vi "AI Test Temp serial v7.vi"(0 "Command String":string, 5 "Time Out (S)":dbl, 7 "CALIB":dbl) -> (4 "T1":dbl, 6 "T2":dbl, 8 "T3":dbl, 10 "T4":dbl, 13 "error":bool, 14 "output cluster":cluster{dbl, dbl, dbl, dbl, i32, "error #":dbl}, 15 "Unit ID":dbl)   [LabVIEW 2013]
panel:
  out "VISA Com out":refnum<visa-resource-name>
  out "Com Port Create loops":i32
  out "Com Port Create":bool
  in  "Select COM port":refnum<visa-resource-name>
  out "error out 1":errorcluster
  in  "Loop Time mS":u32
  in  "stop":bool
  out "error #":dbl
  out "End T":dbl
  out "Start T":dbl
  out "read time":dbl
  in  "Array - String":string[](array[string])
  out "end of data (#)":bool
  out "data bytes read":dbl
  out "data string":string
  out "read buffer":string
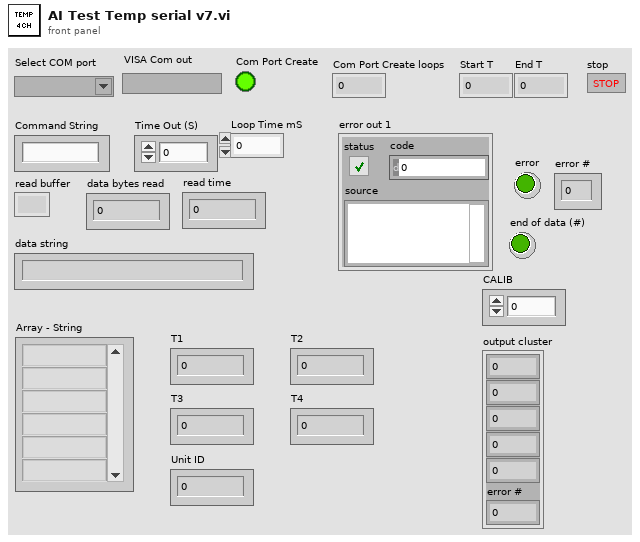
[diagram p1: front panel]
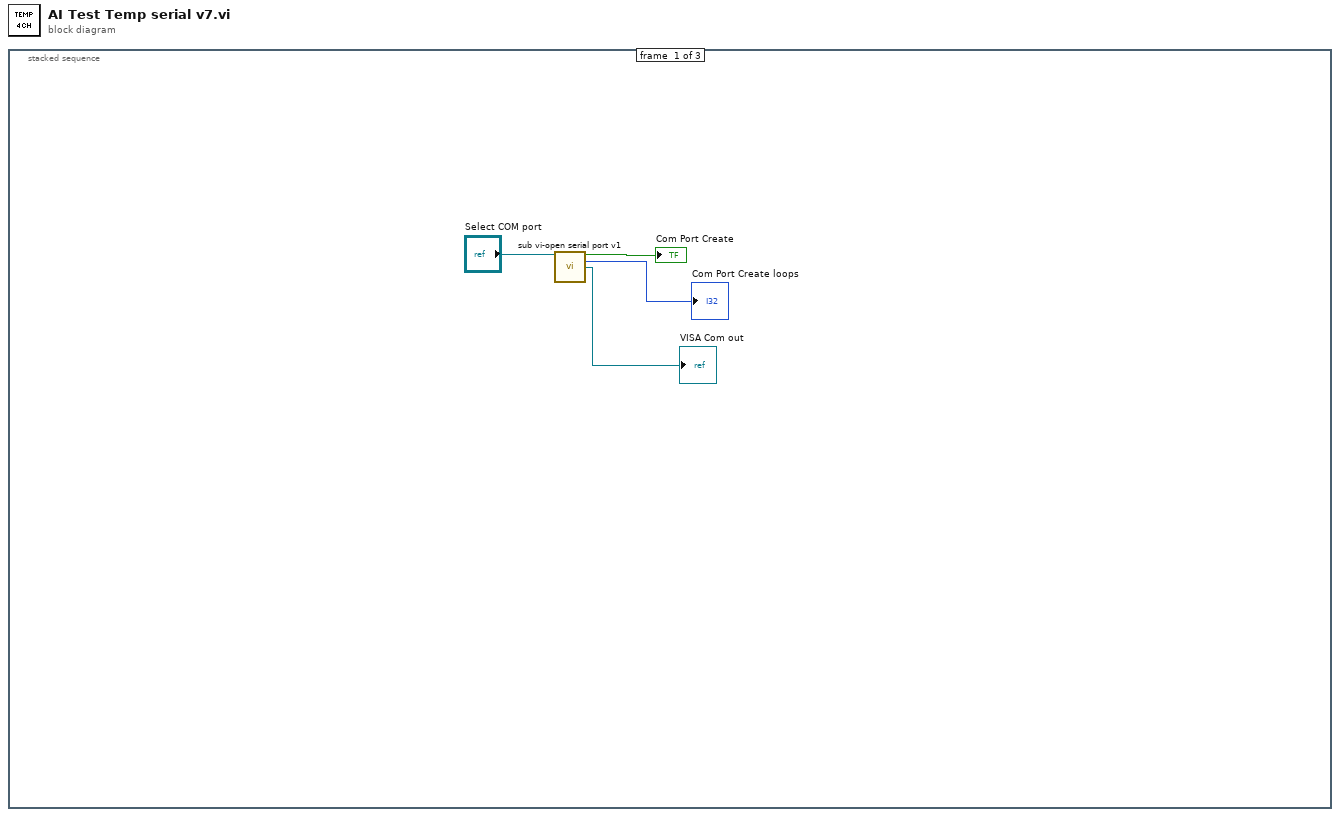
[diagram p0: block diagram]
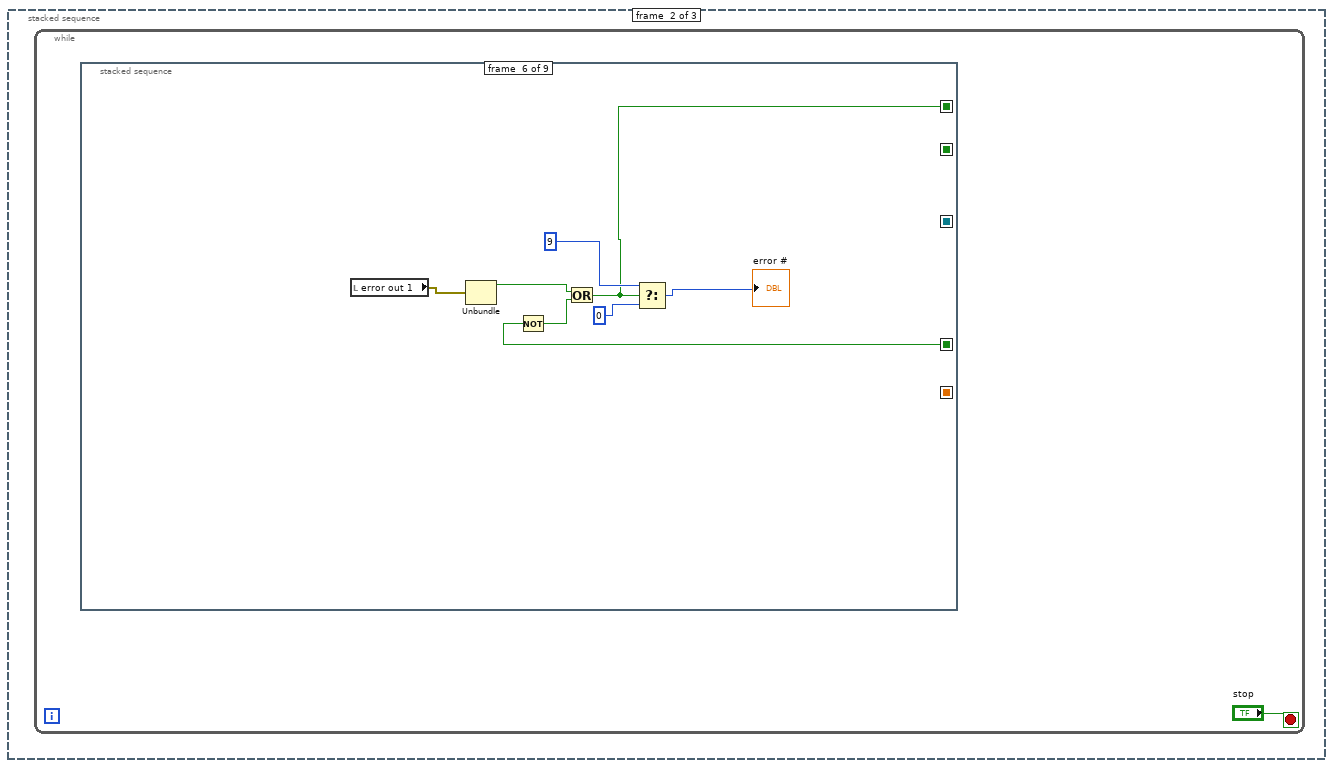
[diagram p2: hidden frame]
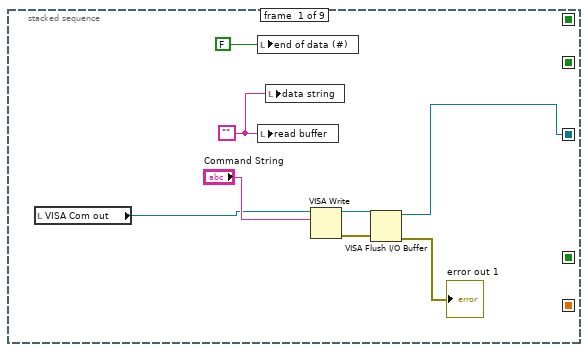
[diagram p3: hidden frame]
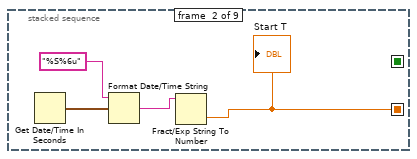
[diagram p4: hidden frame]
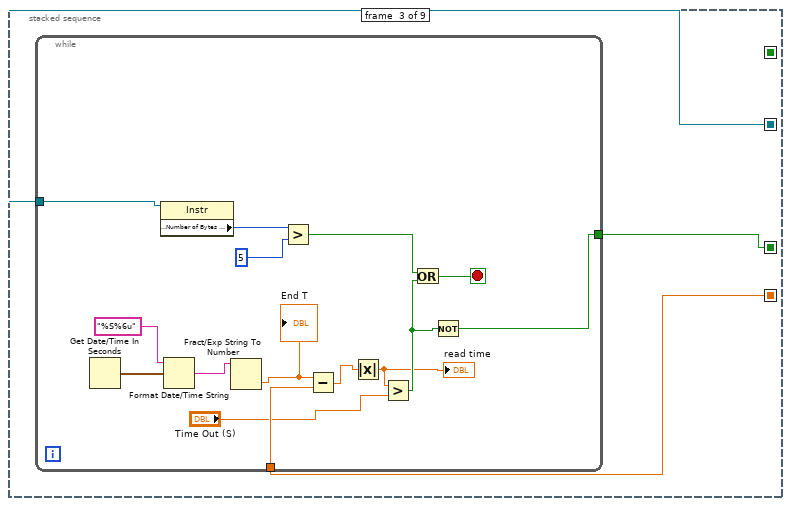
[diagram p5: hidden frame]
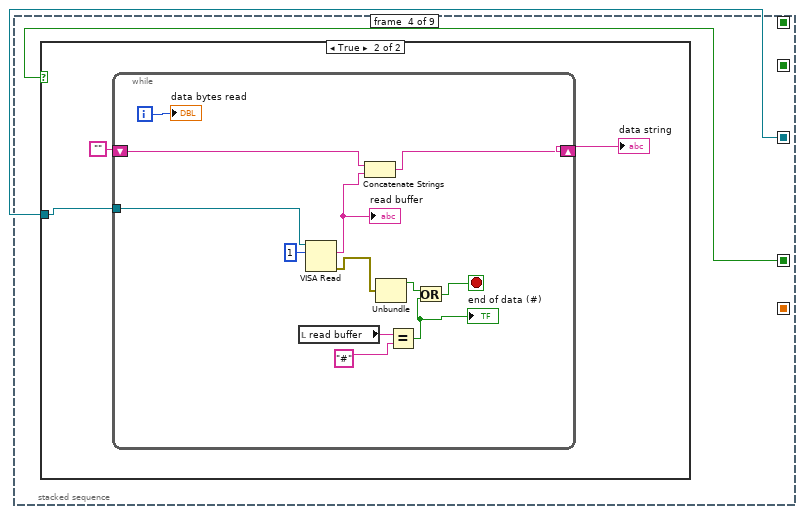
[diagram p6: hidden frame]
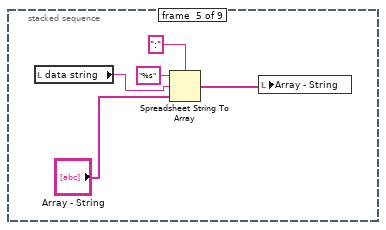
[diagram p8: hidden frame]
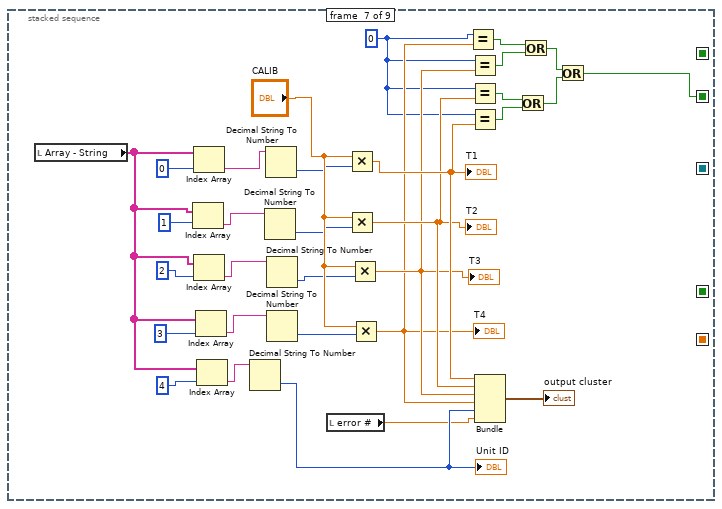
[diagram p9: hidden frame]
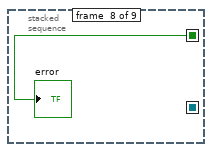
[diagram p10: hidden frame]
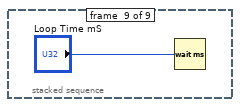
[diagram p11: hidden frame]
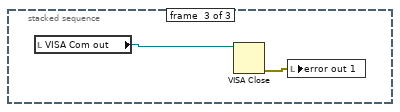
[diagram p12: hidden frame]
diagram:
  n1 = stacked-sequence {
    frame #0 {
      n2 = call "sub vi-open serial port v1.vi"("Select COM port"="Select COM port") -> ("status"=→"Com Port Create":bool, "LOOPS"=→"Com Port Create loops":i32, "VISA Com out"=→"VISA Com out":refnum<visa-resource-name>)  [unwired: 12 in]
    }
    frame #1 {
      n3 = while {
        stop <- "stop" stop-if-true
        n4 = stacked-sequence {
          seq-local: [_ _ w20 _ _ _ _ _ _] -> [_ _ _ w37 _ w65 _ _ _]
          seq-local: [_ w14 _ _ _ _ _ _ _] -> [_ _ w19 _ _ _ _ _ _]
          seq-local: [_ _ _ _ _ w60 _ _ _] -> [_ _ _ _ _ _ _ _ _]
          seq-local: [_ _ _ _ _ _ w66 _ _] -> [_ _ _ _ _ _ _ w97 _]
          seq-local: [w9 _ _ _ _ _ _ _ _] -> [_ _ w18 w36 _ _ _ _ _]
          frame #0 {
            w13 = ""
            n5 = local read "VISA Com out"() -> (w7:refnum<visa-resource-name>)
            n6 = local write "end of data (#)"(FALSE) -> ()
            n7 = local write "read buffer"(w13) -> ()
            n8 = local write "data string"(w13) -> ()
            n9 = VISA Write(VISA resource name=w7, write buffer="Command String") -> (VISA resource name out=w11:refnum<visa-resource-name>, error out=w6:errorcluster)  [unwired: 1 in, 1 out]
            n10 = VISA Flush I/O Buffer(VISA resource name=w11, error in (no error)=w6) -> (VISA resource name out=w9:refnum<visa-resource-name>, error out=→"error out 1":errorcluster)  [unwired: 1 in]
          }
          frame #1 {
            n11 = Get Date/Time In Seconds() -> (seconds since 1Jan1904=w17:timestamp)
            n12 = Format Date/Time String(time format string (%c)="%S%6u", seconds (now)=w17) -> (date/time string=w15:string)  [unwired: 1 in]
            n13 = Fract/Exp String To Number(string=w15) -> (number=w14:dbl)  [unwired: 3 in, 1 out]
            "Start T" <- w14
          }
          frame #2 {
            n14 = while {
              tunnel: w18 -> [w35]
              tunnel: [w24] -> w20
              tunnel: w19 -> [w28]
              stop <- w26 stop-if-true
              n15 = Get Date/Time In Seconds() -> (seconds since 1Jan1904=w32:timestamp)
              n16 = property class="Instr"(reference=w35) -> ("Serial Settings:Number of Bytes at Serial Port"=w34:u32)  [unwired: 1 in, 2 out]
              n17 = Format Date/Time String(time format string (%c)="%S%6u", seconds (now)=w32) -> (date/time string=w30:string)  [unwired: 1 in]
              n18 = Fract/Exp String To Number(string=w30) -> (number=w29:dbl)  [unwired: 3 in, 1 out]
              "End T" <- w29
              n19 = Greater?(x=w34, y=5) -> (0:w27:bool)
              n20 = Subtract(x=w29, y=w28) -> (x-y=w22:dbl)
              n21 = Absolute Value(x=w22) -> (abs(x)=w21:dbl)
              "read time" <- w21
              n22 = Greater?(x=w21, y="Time Out (S)") -> (0:w25:bool)
              n23 = Or(x=w27, y=w25) -> (x .or. y?=w26:bool)
              n24 = Not(x=w25) -> (.not. x?=w24:bool)
            }
          }
          frame #3 {
            n25 = case shown="True" w37 {
              tunnel: w36 -> [_ w40]
              frame False {
              }
              frame True {
                n26 = while {
                  tunnel: w40 -> [w47]
                  shift-right: [w46] -> w39
                  shift-left: "" -> [w45]
                  i -> [w48]
                  stop <- w41 stop-if-true
                  n27 = local read "read buffer"() -> (w51:string)
                  n28 = VISA Read(VISA resource name=w47, byte count=u32 1) -> (read buffer=w49:string, error out=w44:errorcluster)  [unwired: 1 in, 2 out]
                  "read buffer" <- w49
                  n29 = Concatenate Strings(w45, w49) -> (w46:string)
                  n30 = Unbundle(w44) -> ("status"=w43:bool)  [unwired: 2 out]
                  n31 = Equal?(x=w51, y="#") -> (x = y?=w42:bool)
                  "end of data (#)" <- w42
                  n32 = Or(x=w43, y=w42) -> (x .or. y?=w41:bool)
                  "data bytes read" <- w48
                }
                "data string" <- w39
              }
            }
          }
          frame #4 {
            n33 = local read "data string"() -> (w55:string)
            n34 = Spreadsheet String To Array(delimiter (Tab)=":", format string="%s", spreadsheet string=w55, array type (2D Dbl)="Array - String") -> (array=w53:string[])
            n35 = local write "Array - String"(w53) -> ()
          }
          frame #5 {
            n36 = local read "error out 1"() -> (w59:errorcluster)
            n37 = Unbundle(w59) -> ("status"=w58:bool)  [unwired: 2 out]
            n38 = Not(x=w65) -> (.not. x?=w64:bool)
            n39 = Or(x=w58, y=w64) -> (x .or. y?=w60:bool)
            n40 = Select(t=9, s=w60, f=0) -> (s? t:f=→"error #":i32)
          }
          frame #6 {
            w73 = 0
            n41 = local read "Array - String"() -> (w88:string[])
            n42 = Index Array(array=w88, index=1) -> (element=w91:string)
            n43 = Index Array(array=w88, index=0) -> (element=w95:string)
            n44 = Index Array(array=w88, index=2) -> (element=w90:string)
            n45 = Index Array(array=w88, index=3) -> (element=w89:string)
            n46 = Index Array(array=w88, index=4) -> (element=w86:string)
            n47 = Decimal String To Number(string=w86) -> (number=w80:i32)  [unwired: 2 in, 1 out]
            "Unit ID" <- w80
            n48 = Decimal String To Number(string=w91) -> (number=w83:i32)  [unwired: 2 in, 1 out]
            n49 = Decimal String To Number(string=w95) -> (number=w84:i32)  [unwired: 2 in, 1 out]
            n50 = Decimal String To Number(string=w90) -> (number=w82:i32)  [unwired: 2 in, 1 out]
            n51 = Decimal String To Number(string=w89) -> (number=w81:i32)  [unwired: 2 in, 1 out]
            n52 = local read "error #"() -> (w79:dbl)
            n53 = Multiply(x="CALIB", y=w84) -> (x*y=w77:dbl)
            "T1" <- w77
            n54 = Multiply(x="CALIB", y=w83) -> (x*y=w76:dbl)
            "T2" <- w76
            n55 = Multiply(x="CALIB", y=w82) -> (x*y=w75:dbl)
            "T3" <- w75
            n56 = Multiply(x="CALIB", y=w81) -> (x*y=w74:dbl)
            "T4" <- w74
            n57 = Equal?(x=w73, y=w74) -> (x = y?=w69:bool)
            n58 = Equal?(x=w73, y=w75) -> (x = y?=w70:bool)
            n59 = Equal?(x=w73, y=w76) -> (x = y?=w72:bool)
            n60 = Equal?(x=w73, y=w77) -> (x = y?=w71:bool)
            n61 = Bundle(w77, w76, w75, w74, w80, "error #"=w79) -> (→"output cluster":cluster{dbl, dbl, dbl, dbl, i32, "error #":dbl})  [unwired: 1 in]
            n62 = Or(x=w72, y=w71) -> (x .or. y?=w67:bool)
            n63 = Or(x=w69, y=w70) -> (x .or. y?=w68:bool)
            n64 = Or(x=w68, y=w67) -> (x .or. y?=w66:bool)
          }
          frame #7 {
            "error" <- w97
          }
          frame #8 {
            n65 = Wait (ms)(milliseconds to wait="Loop Time mS") -> ()  [unwired: 1 out]
          }
        }
      }
    }
    frame #2 {
      n66 = local read "VISA Com out"() -> (w100:refnum<visa-resource-name>)
      n67 = VISA Close(VISA resource name=w100) -> (error out=w99:errorcluster)  [unwired: 1 in]
      n68 = local write "error out 1"(w99) -> ()
    }
  }
